vi "JSR Init.vi"(8 "error in (no error)":errorcluster, 10 "Pulser State (T: ON)":bool=TRUE, 11 "JSR VISA":refnum<visa-resource-name>="COM4") -> (0 "error out":errorcluster, 3 "JSR VISA Out":refnum<visa-resource-name>)   [LabVIEW 2022 SP3]
uses:
  PulserGlobals.vi
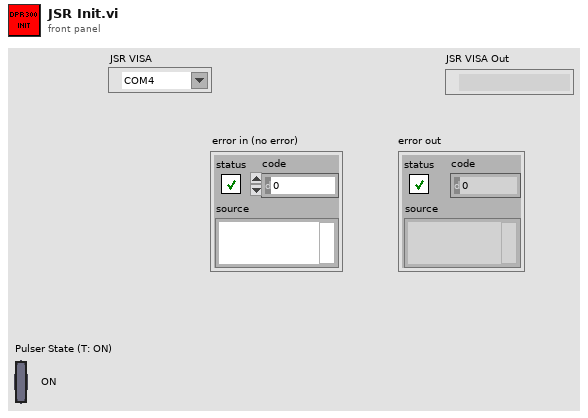
[diagram p1: front panel]
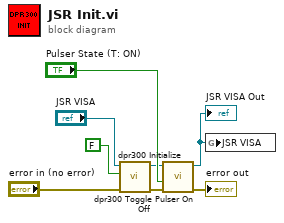
[diagram p0: block diagram]
diagram:
  n1 = call <instrlib>:"dpr300 Initialize.vi"("error in (no error)"="error in (no error)", "ID Query? (T: Yes)"=FALSE, "VISA resource name"="JSR VISA") -> ("error out"=w3:errorcluster, "VISA resource name out"=w4:refnum<visa-resource-name>)  [unwired: 6 in, 1 out]
  n2 = call <instrlib>:"dpr300 Toggle Pulser On Off.vi"("error in (no error)"=w3, "Pulser State (T: ON)"="Pulser State (T: ON)", "VISA resource name"=w4) -> ("error out"=→"error out":errorcluster, "VISA resource name out"=w2:refnum<visa-resource-name>)  [unwired: 7 in]
  "JSR VISA Out" <- w2
  n3 = global write "PulserGlobals.vi" "JSR VISA"(w2) -> ()
